vi "gate voltage header.vi"() -> (0 "Array":string[][](array[string]))   [LabVIEW 2021]
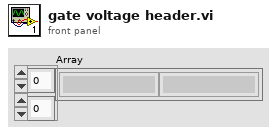
[diagram p1: front panel]
types:
  T1 = enum16{"Set Voltage", "Read Voltage", "Read Setpoint", "Read Current", "Output On", "Output Off"}
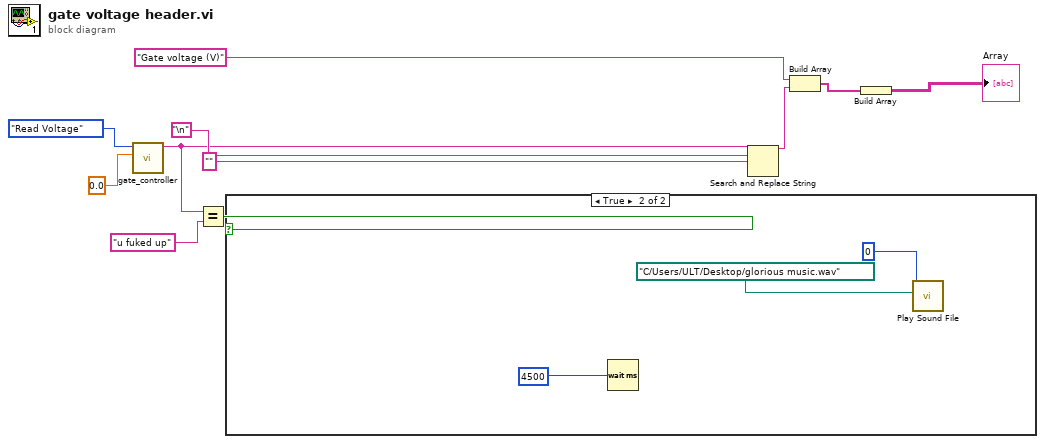
[diagram p0: block diagram]
diagram:
  n1 = call "gate_controller.vi"("Numerical Argument"=0.0, "Command"=T1."Read Voltage") -> ("Response"=w2:string)  [unwired: 9 in]
  n2 = Equal?(x=w2, y="u fuked up") -> (x = y?=w1:bool)
  n3 = case shown="True" w1 {
    frame False {
    }
    frame True {
      n4 = Wait (ms)(milliseconds to wait=u32 4500) -> ()  [unwired: 1 out]
      n5 = call <vilib>:"Play Sound File.vi"("path"=path "C:/Users/ULT/Desktop/glorious music.wav", "device ID"=u32 0) -> ()  [unwired: 8 in, 2 out]
    }
  }
  n6 = Search and Replace String(input string=w2, search string="\n", replace string="" ("replace string (\"\")")) -> (result string=w4:string)  [unwired: 5 in, 3 out]
  n7 = Build Array("Gate voltage (V)", w4) -> (w8:string[])
  n8 = Build Array(w8) -> (→"Array":string[][])
